vi "总氮质控流程.vi"(6 "队列输入TN":refnum<queue>, 9 "总氮":bool, 10 "总氮量程切换":enum32{"H", "L", "AUTO"}(ring)=enum."AUTO") -> (3 "布尔":bool)   [LabVIEW 2016, in "质控单元.lvlib"]
panel:
  out "总氮中断报警":bool
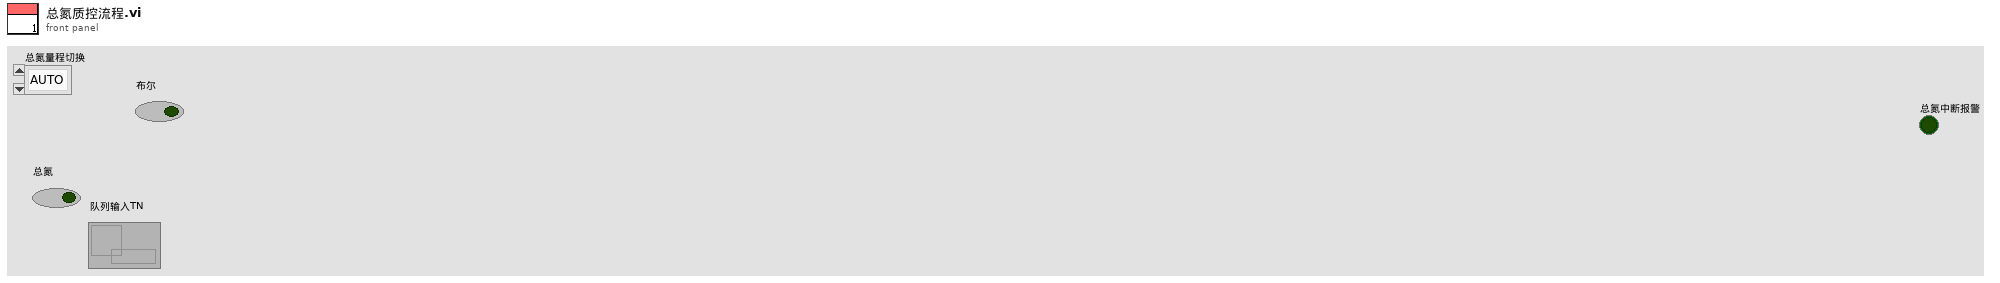
[diagram p1: front panel]
types:
  T1 = enum16{"待机", "启动氨氮水样", "氨氮测量中", "启动氨氮加标", "启动氨氮加标回收", "氨氮加标回收测量中", "启动总氮水样", "总氮测量中", "启动总氮加标", "启动总氮加标回收", "总氮加标回收测量中", "启动总磷水样", "总磷水样测量中", "启动总磷加标", "启动总磷加标回收", "总磷加标回收测量中", "结束"}
  T2 = cluster{"站号":u16, "量程切换":enum32{"H", "L", "AUTO"}, "控制命令":enum16{"启动测量", "标样核查", "零点核查", "跨度核查", "空白测试", "平行样测试", "加标回收", "空白校准", "标样校准", "初始化（清洗）", "停止测试", "仪器重启", "校时", "模式设置", "测量间隔设置"}, "模式设置":enum16{"待机", "连续模式", "周期模式", "定点模式", "受控模式", "手动模式"}, "测量间隔":u16}
  T3 = cluster{"时间标识":timestamp, "设备":string, "日志信息":string}
  T4 = cluster{"系统时间":timestamp, "工作状态":enum16{"空闲", "水样测试", "标样核查", "零点核查", "跨度核查", "空白测试", "平行样测试", "加标回收", "空白校准", "标样校准", "初始化（清洗）"}, "测量模式":enum16{"待机", "连续模式", "周期模式", "定点模式", "受控模式", "手动模式"}, "告警代码":enum16{"无告警", "缺试剂告警", "缺水样告警", "缺蒸馏水告警", "缺标液告警", "仪表漏液告警", "标定异常告警", "超量程告警", "加热异常", "低试剂预警", "超上限告警", "超下限告警", "仪表内部其他异常", "滴定异常告警", "电极异常告警", "量程切换告警", "参数设置告警", "PH电极电位异常", "电导率电极异常", "浊度光度异常", "溶解氧电极异常", "溶解氧光强异常", "温度异常告警", "PH异常告警", "溶解氧异常告警", "电导率异常告警", "浊度异常告警", "叶绿素异常告警", "藻密度异常告警", "蓝绿藻异常告警", "ORP异常告警", "氨氮异常告警", "清洁刷异常告警", "SD卡异常告警", "蓝牙异常告警", "Wifi异常告警", "流程异常告警"}, "故障代码":enum16{"无故障", "电机故障", "温度故障", "通讯故障", "滴定故障"}, "日志代码":u16, "软件版本":u16, "F0":sgl, "F1":sgl, "F2":sgl, "F3":sgl, "T":sgl, "H":sgl, "id":u16, "flowid":u16, "量程":u16, "总磷控温温度1":sgl, "营养盐控温温度2":sgl, "ADC":sgl}
  T5 = enum16{"空闲", "水样测试", "标样核查", "零点核查", "跨度核查", "空白测试", "平行样测试", "加标回收", "空白校准", "标样校准", "初始化（清洗）"}
  T6 = cluster{"因子编码":u32, "单位":u16, "标样参考值":sgl, "水样数据时间":timestamp, "水样实测值":sgl, "水样数据标识":string, "标样数据时间":timestamp, "标样实测值":sgl, "标样数据标识":string, "空白数据时间":timestamp, "空白实测值":sgl, "空白数据标识":string, "零点核查数据时间":timestamp, "零点核查实测值":sgl, "零点核查数据标识":string, "跨度核查数据时间":timestamp, "跨度核查实测值":sgl, "跨度核查数据标识":string, "加标回收数据时间":timestamp, "加标回收实测值":sgl, "加标回收数据标识":string, "平行样数据时间":timestamp, "平行样实测值":sgl, "平行样数据标识":string}
  T7 = cluster{"量程":dbl, "检出限":dbl, "加标前水样浓度":dbl, "加标后水样浓度":dbl, "加标水杯定容体积":dbl, "加标母液浓度":dbl, "加标体积":dbl, "加标回收率":dbl}
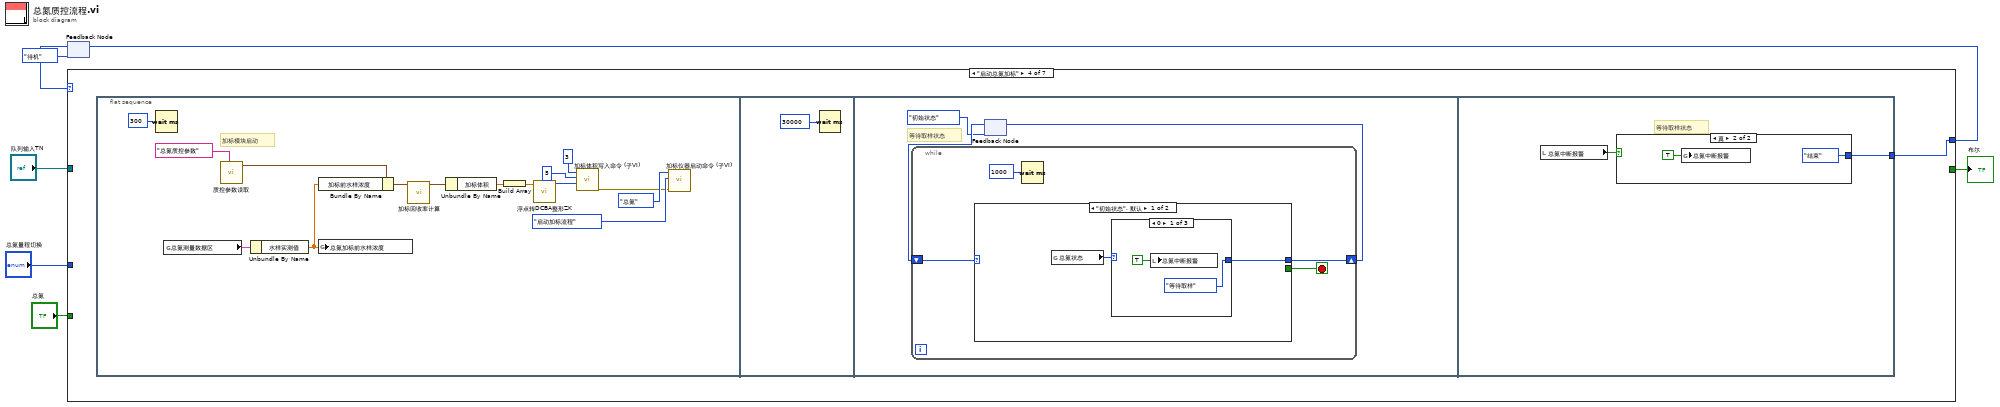
[diagram p0: block diagram]
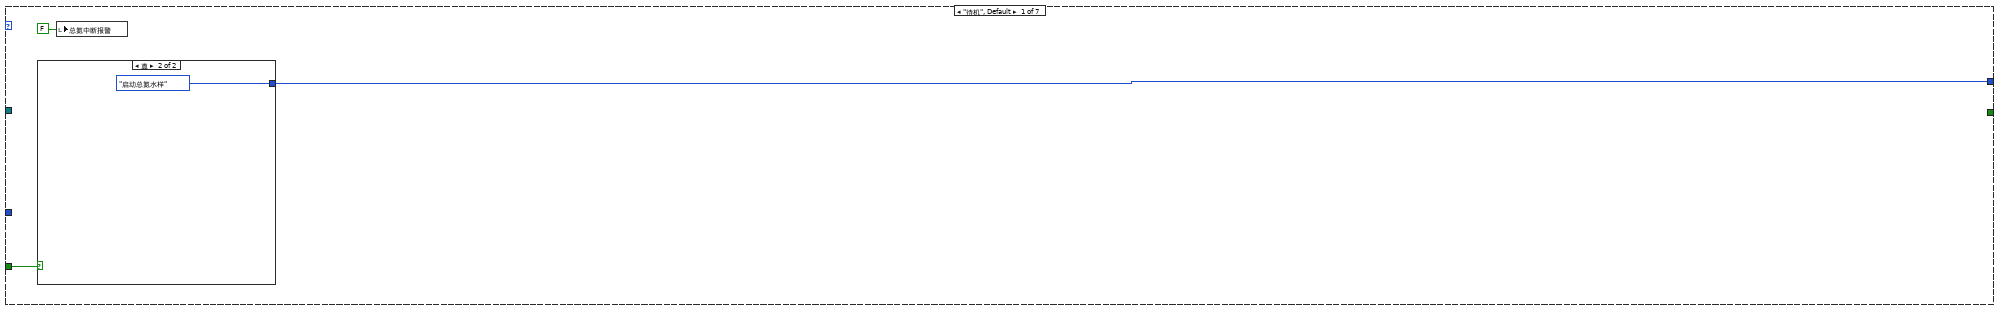
[diagram p2: hidden frame]
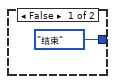
[diagram p3: hidden frame]
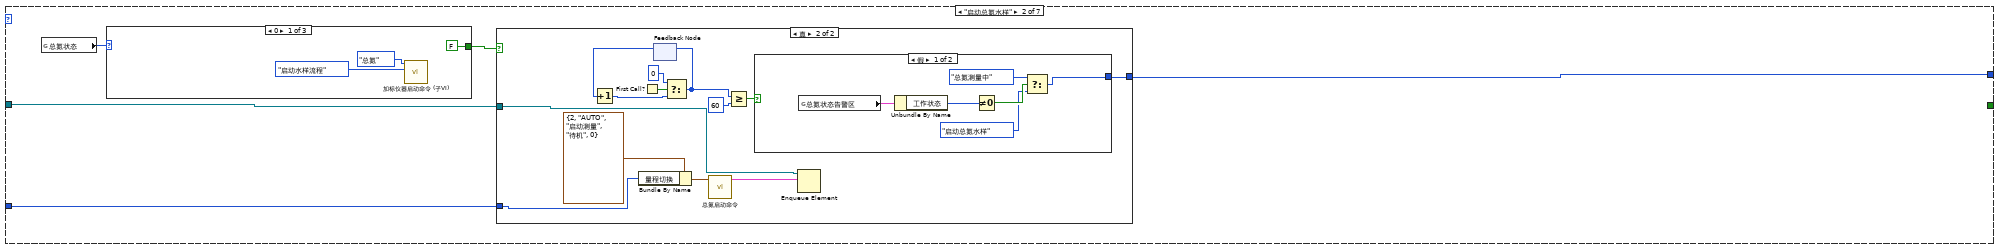
[diagram p4: hidden frame]
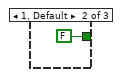
[diagram p5: hidden frame]
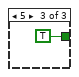
[diagram p6: hidden frame]
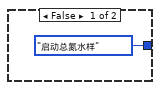
[diagram p7: hidden frame]
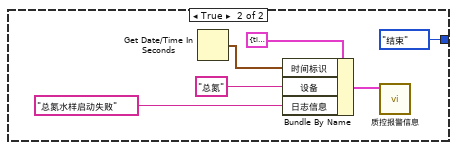
[diagram p8: hidden frame]
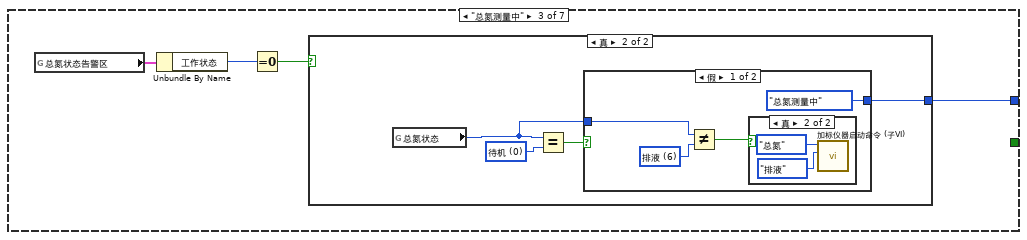
[diagram p9: hidden frame]
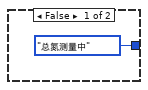
[diagram p10: hidden frame]
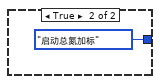
[diagram p12: hidden frame]
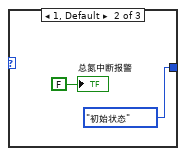
[diagram p13: hidden frame]
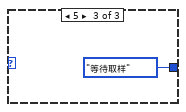
[diagram p14: hidden frame]
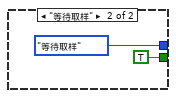
[diagram p15: hidden frame]
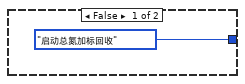
[diagram p16: hidden frame]
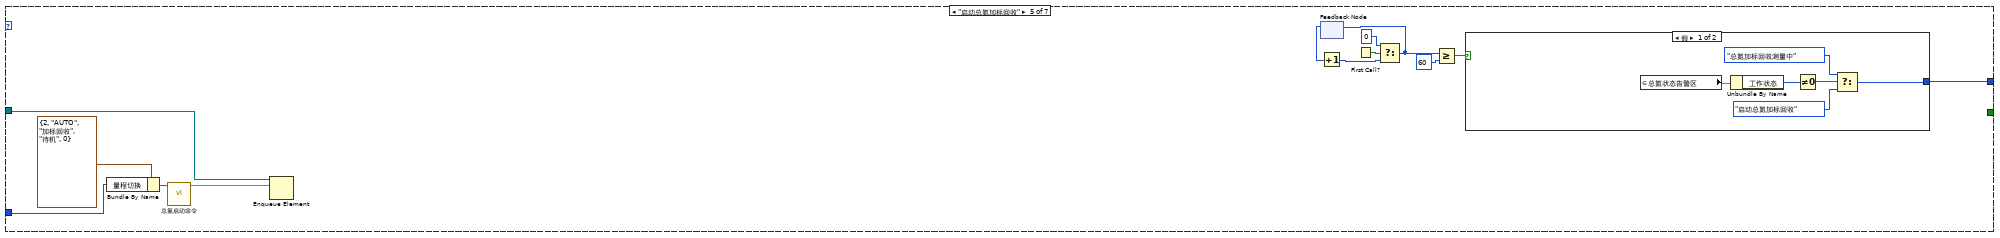
[diagram p17: hidden frame]
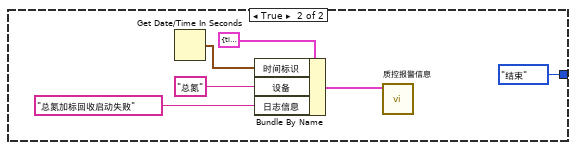
[diagram p18: hidden frame]
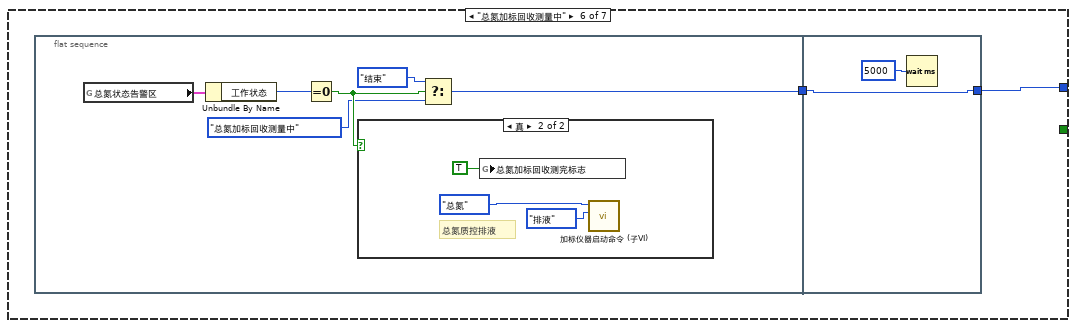
[diagram p19: hidden frame]
diagram:
  n1 = feedback #1(T1."待机") -> (w5:T1)
  n2 = case shown="\"启动总氮加标\"" w5 {
    tunnel: [w10 w17 w49 w65 w108 w128 T1."结束"] -> w3
    tunnel: [_ _ _ _ _ _ TRUE] -> w6
    tunnel: "总氮" -> [w9 _ _ _ _ _ _]
    tunnel: "队列输入TN" -> [_ w16 _ _ w107 _ _]
    tunnel: "总氮量程切换" -> [_ w15 _ _ w104 _ _]
    frame "待机", Default {
      n3 = case shown="真" w9 {
        tunnel: [T1."结束" T1."启动总氮水样"] -> w10
        frame False {
        }
        frame True {
        }
      }
      n4 = local write "总氮中断报警"(FALSE ("氨氮中断报警")) -> ()
    }
    frame "启动总氮水样" {
      n5 = global read "加标回收状态全局变量.vi" "总氮状态"() -> (w14:u16)
      n6 = case shown="0" w14 {
        tunnel: [FALSE ("s") FALSE ("s") TRUE ("s")] -> w13
        frame 0 {
          n7 = call "加标仪器启动命令 (子VI).vi"("启动命令"=enum16{"启动水样流程", "启动加标流程", "排液", "停止"}."启动水样流程", "仪器"=enum16{"", "氨氮", "总磷", "总氮", "CODMn", "CODCr"}."总氮") -> ()  [unwired: 9 in, 1 out]
        }
        frame 1, Default {
        }
        frame 5 {
        }
      }
      n8 = case shown="真" w13 {
        tunnel: [T1."启动总氮水样" w36] -> w17
        tunnel: w16 -> [_ w28]
        tunnel: w15 -> [_ w25]
        frame False {
        }
        frame True {
          n9 = Bundle By Name(cluster=T2 {"站号"=2, "量程切换"=enum."AUTO", "控制命令"=enum."启动测量", "模式设置"=enum."待机", "测量间隔"=0} ("参数"), "量程切换"=w25) -> (w27:T2)
          n10 = First Call?() -> (First Call?: T/F=w34:bool)
          n11 = feedback #2() -> (w33:i32)  [unwired: 1 in]
          n12 = Increment(x=w33) -> (x+1=w32:i32)
          n13 = Select(t=0, s=w34, f=w32) -> (s? t:f=w31:i32)
          n14 = feedback-in #2(w31) -> ()
          n15 = call "总氮启动命令.vi"("参数"=w27) -> ("启动命令"=w24:cluster{"命令":string, "data":variant})  [unwired: 10 in]
          n16 = Greater Or Equal?(x=w31, y=60) -> (x >= y?=w29:bool)
          n17 = case shown="假" w29 {
            tunnel: [w41 T1."结束"] -> w36
            frame False {
              n18 = global read "与总氮交互全局.vi" "总氮状态告警区"() -> (w38:T4)
              n19 = Unbundle By Name(w38) -> ("工作状态"=w37:T5)
              n20 = Not Equal To 0?(x=w37) -> (x != 0?=w42:bool)
              n21 = Select(t=T1."总氮测量中", s=w42, f=T1."启动总氮水样") -> (s? t:f=w41:T1)
            }
            frame True {
              n22 = Get Date/Time In Seconds() -> (seconds since 1Jan1904=w48:timestamp)
              n23 = Bundle By Name(cluster=T3 {"时间标识"=timestamp(0 s since 1904-01-01), "设备"="", "日志信息"=""} ("data in"), "时间标识"=w48, "设备"="总氮", "日志信息"="总氮水样启动失败") -> (w43:T3)
              n24 = call "质控报警信息.vi"("data in"=w43) -> ()  [unwired: 10 in, 1 out]
            }
          }
          n25 = Enqueue Element(queue=w28, element=w24) -> ()  [unwired: 2 in, 3 out]
        }
      }
    }
    frame "总氮测量中" {
      n26 = global read "与总氮交互全局.vi" "总氮状态告警区"() -> (w52:T4)
      n27 = Unbundle By Name(w52) -> ("工作状态"=w50:T5)
      n28 = Equal To 0?(x=w50) -> (x = 0?=w51:bool)
      n29 = case shown="真" w51 {
        tunnel: [T1."总氮测量中" w55] -> w49
        frame False {
        }
        frame True {
          w57 = u16 0 items=["待机", "润洗", "进样", "进样完成", "柱塞泵加标", "等待取液", "排液"] ("氨氮状态")
          n30 = global read "加标回收状态全局变量.vi" "总氮状态"() -> (w54:u16)
          n31 = Equal?(x=w54, y=w57) -> (x = y?=w56:bool)
          n32 = case shown="假" w56 {
            tunnel: [T1."总氮测量中" T1."启动总氮加标"] -> w55
            tunnel: w54 -> [w58 _]
            frame False {
              w60 = u16 6 items=["待机", "润洗", "进样", "进样完成", "柱塞泵加标", "等待取液", "排液"] ("氨氮状态")
              n33 = Not Equal?(x=w58, y=w60) -> (x != y?=w59:bool)
              n34 = case shown="真" w59 {
                frame False {
                }
                frame True {
                  n35 = call "加标仪器启动命令 (子VI).vi"("启动命令"=enum16{"启动水样流程", "启动加标流程", "排液", "停止"}."排液", "仪器"=enum16{"", "氨氮", "总磷", "总氮", "CODMn", "CODCr"}."总氮") -> ()  [unwired: 9 in, 1 out]
                }
              }
            }
            frame True {
            }
          }
        }
      }
    }
    frame "启动总氮加标" {
      n36 = flat-sequence {
        tunnel: [w99] -> w65
        frame #0 {
          # "加标模块启动"
          n37 = Wait (ms)(milliseconds to wait=u32 300 ("等待时间（毫秒）")) -> ()  [unwired: 1 out]
          n38 = global read "与总氮交互全局.vi" "总氮测量数据区"() -> (w73:T6)
          n39 = call "质控参数读取.vi"("section"="总氮质控参数") -> ("参数"=w78:T7)  [unwired: 9 in, 1 out]
          n40 = Unbundle By Name(w73) -> ("水样实测值"=w75:sgl)
          n41 = Bundle By Name(cluster=w78, "加标前水样浓度"=w75) -> (w79:T7)
          n42 = global write "水样浓度全局.vi" "总氮加标前水样浓度"(w75) -> ()
          n43 = call "加标回收率计算.vi"("参数"=w79) -> ("参数 out"=w77:T7)  [unwired: 10 in]
          n44 = Unbundle By Name(w77) -> ("加标体积"=w76:dbl)
          n45 = Build Array(w76) -> (w72:dbl[])
          n46 = call "浮点转DCBA整形ZK.vi"("浮点数"=w72) -> ("DCBA整形输出"=w67:u16[])  [unwired: 10 in]
          n47 = call "加标体积写入命令 (子VI).vi"("values"=w67, "starting address"=u16 5, "Slave ID"=u16 3 ("value")) -> ("错误输出"=w66:errorcluster)  [unwired: 8 in]
          n48 = call "加标仪器启动命令 (子VI).vi"("错误输入（无错误）"=w66, "启动命令"=enum16{"启动水样流程", "启动加标流程", "排液", "停止"}."启动加标流程", "仪器"=enum16{"", "氨氮", "总磷", "总氮", "CODMn", "CODCr"}."总氮") -> ()  [unwired: 8 in, 1 out]
        }
        frame #1 {
          n49 = Wait (ms)(milliseconds to wait=u32 30000 ("等待时间（毫秒）")) -> ()  [unwired: 1 out]
        }
        frame #2 {
          # "等待取样状态"
          n50 = feedback #3(enum16{"初始状态", "等待取样"}."初始状态") -> (w83:enum16{"初始状态", "等待取样"})
          n51 = while {
            shift-right: [w87] -> w84
            shift-left: w83 -> [w88]
            stop <- w86 stop-if-true
            n52 = case shown="\"初始状态\", 默认" w88 {
              tunnel: [w90 enum16{"初始状态", "等待取样"}."等待取样"] -> w87
              tunnel: [_ TRUE] -> w86
              frame "初始状态", Default {
                n53 = global read "加标回收状态全局变量.vi" "总氮状态"() -> (w89:u16)
                n54 = case shown="0" w89 {
                  tunnel: [enum16{"初始状态", "等待取样"}."等待取样" enum16{"初始状态", "等待取样"}."初始状态" enum16{"初始状态", "等待取样"}."等待取样"] -> w90
                  frame 0 {
                    n55 = local write "总氮中断报警"(TRUE ("氨氮中断报警")) -> ()
                  }
                  frame 1, Default {
                    "总氮中断报警" <- FALSE ("总氮中断报警")
                  }
                  frame 5 {
                  }
                }
              }
              frame "等待取样" {
              }
            }
            n56 = Wait (ms)(milliseconds to wait=u32 1000 ("等待时间（毫秒）")) -> ()  [unwired: 1 out]
          }
          n57 = feedback-in #3(w84) -> ()
        }
        frame #3 {
          # "等待取样状态"
          n58 = local read "总氮中断报警"() -> (w98:bool)
          n59 = case shown="真" w98 {
            tunnel: [T1."启动总氮加标回收" T1."结束"] -> w99
            frame False {
            }
            frame True {
              n60 = global write "质控中断报警全局.vi" "总氮中断报警"(TRUE ("总氮中断报警")) -> ()
            }
          }
        }
      }
    }
    frame "启动总氮加标回收" {
      n61 = Bundle By Name(cluster=T2 {"站号"=2, "量程切换"=enum."AUTO", "控制命令"=enum."加标回收", "模式设置"=enum."待机", "测量间隔"=0} ("参数"), "量程切换"=w104) -> (w106:T2)
      n62 = call "总氮启动命令.vi"("参数"=w106) -> ("启动命令"=w103:cluster{"命令":string, "data":variant})  [unwired: 10 in]
      n63 = Enqueue Element(queue=w107, element=w103) -> ()  [unwired: 2 in, 3 out]
      n64 = feedback #4() -> (w113:i32)  [unwired: 1 in]
      n65 = Increment(x=w113) -> (x+1=w112:i32)
      n66 = First Call?() -> (First Call?: T/F=w114:bool)
      n67 = Select(t=0, s=w114, f=w112) -> (s? t:f=w111:i32)
      n68 = feedback-in #4(w111) -> ()
      n69 = Greater Or Equal?(x=w111, y=60) -> (x >= y?=w109:bool)
      n70 = case shown="假" w109 {
        tunnel: [w119 T1."结束"] -> w108
        frame False {
          n71 = global read "与总氮交互全局.vi" "总氮状态告警区"() -> (w116:T4)
          n72 = Unbundle By Name(w116) -> ("工作状态"=w121:T5)
          n73 = Not Equal To 0?(x=w121) -> (x != 0?=w120:bool)
          n74 = Select(t=T1."总氮加标回收测量中", s=w120, f=T1."启动总氮加标回收") -> (s? t:f=w119:T1)
        }
        frame True {
          n75 = Get Date/Time In Seconds() -> (seconds since 1Jan1904=w127:timestamp)
          n76 = Bundle By Name(cluster=T3 {"时间标识"=timestamp(0 s since 1904-01-01), "设备"="", "日志信息"=""} ("data in"), "时间标识"=w127, "设备"="总氮", "日志信息"="总氮加标回收启动失败") -> (w122:T3)
          n77 = call "质控报警信息.vi"("data in"=w122) -> ()  [unwired: 10 in, 1 out]
        }
      }
    }
    frame "总氮加标回收测量中" {
      n78 = flat-sequence {
        tunnel: [w134] -> w129
        tunnel: [w140] -> w128
        tunnel: w129 -> [w140]
        frame #0 {
          n79 = global read "与总氮交互全局.vi" "总氮状态告警区"() -> (w130:T4)
          n80 = Unbundle By Name(w130) -> ("工作状态"=w135:T5)
          n81 = Equal To 0?(x=w135) -> (x = 0?=w132:bool)
          n82 = case shown="真" w132 {
            frame False {
            }
            frame True {
              # "总氮质控排液"
              n83 = global write "质控测完标志全局 1.vi" "总氮加标回收测完标志"(TRUE) -> ()
              n84 = call "加标仪器启动命令 (子VI).vi"("启动命令"=enum16{"启动水样流程", "启动加标流程", "排液", "停止"}."排液", "仪器"=enum16{"", "氨氮", "总磷", "总氮", "CODMn", "CODCr"}."总氮") -> ()  [unwired: 9 in, 1 out]
            }
          }
          n85 = Select(t=T1."结束", s=w132, f=T1."总氮加标回收测量中") -> (s? t:f=w134:T1)
        }
        frame #1 {
          n86 = Wait (ms)(milliseconds to wait=u32 5000 ("等待时间（毫秒）")) -> ()  [unwired: 1 out]
        }
      }
    }
    frame "结束" {
    }
  }
  "布尔" <- w6
  n87 = feedback-in #1(w3) -> ()
